vi "Verify Account Number.vi"(8 "error in":errorcluster, 11 "Module Data":T1={"UI Controls"={"ATM Messages"=refnum, "User Input"=refnum, "Right Buttons"=refnum, "Right Menu"=refnum, "Left Buttons"=refnum, "Left Menu"=refnum, "Card Simulator"=refnum, "Enter"=refnum}, "ATM Messages 2"={"Session terminate message"="Your session has been terminated\ndue to inactivity or menu selection.\nPlease take your card\n\nGoodbye!", "Welcome message"="Welcome to Acme bank.\nPlease insert your card\nand enter your account\nnumber in the User Input.\n\nPress Enter (E) when done.", "Deposit Message"="Please enter amount to deposit and press\nEnter (E) when done.", "Deposit Complete Message"="$ (Amount) Deposited", "Withdrawal Message"="Please enter amount to withdraw and press\nEnter (E) when done.", "Withdrawal Complete Message"="$ (Amount) Withdrawn", "Balance Inquiry Message"="Your Balance Is:\n$ (Balance amount from file)", "Account verification failed message"="Account information incorrect\nPlease Re-Enter Account Number.\nPress Enter (E) when done.", "Withdrawal failed message"="Insufficient funds in account\nplease check your balance\nand try again", "Card Inserted"="Card Inserted", "Main Menu message"="Welcome to Acme bank.\nFirst name, last Name (from file)\n\nplease select transaction\nby using the buttons."}, "User Input"="", "ATM Messages"="", "Acc. file path"=path "", "Accounts Data"=[], "User Input Data"={"Account No"="", "Amount"="", "Activity"=enum."Fast Cash $50"}, "Message"=""}) -> (0 "error out":errorcluster, 1 "Accounts all data":string[][](array[string]), 2 "Index account no.":i32, 3 "Is account?":bool, 4 "Balances Column":string[](array[string]))   [LabVIEW 2016]
doc: "Verify if user account exist and index account number."
uses:
  Controls/UI Controls.ctl
  Controls/ATM Messages.ctl
  Controls/Module Data.ctl
  Controls/User Input Data.ctl
  Controls/Transaction Status.ctl
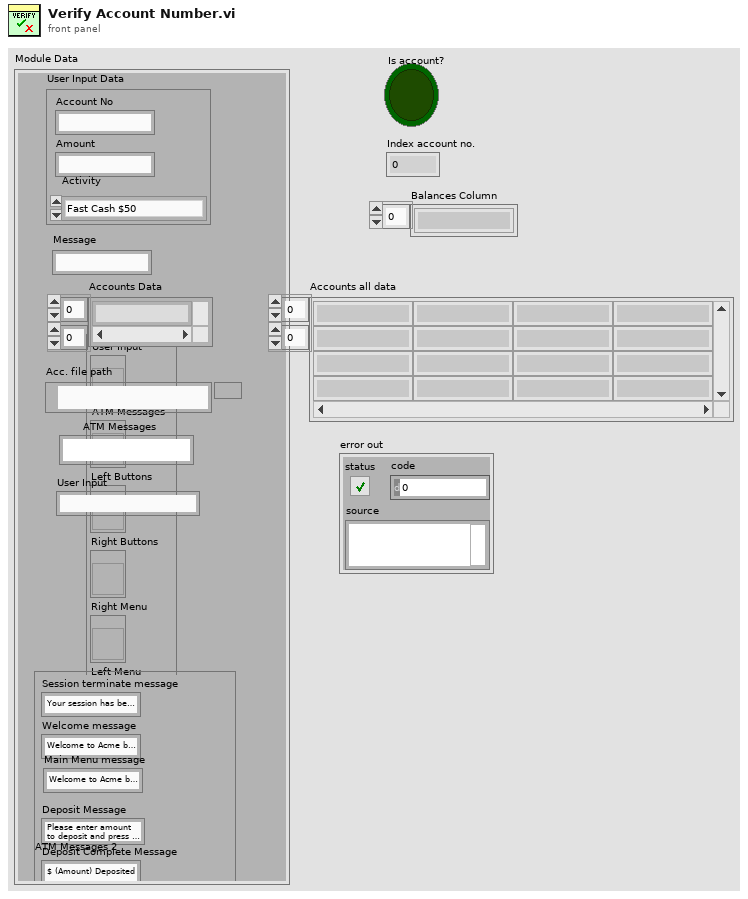
[diagram p1: front panel]
types:
  T1 = typedef "Module Data.ctl" = cluster{"UI Controls":T2, "ATM Messages 2":T3, "User Input":string, "ATM Messages":string, "Acc. file path":path, "Accounts Data":string[][], "User Input Data":T4, "Message":string}
  T2 = typedef "UI Controls.ctl" = cluster{"ATM Messages":refnum<vi>, "User Input":refnum<vi>, "Right Buttons":refnum<vi>, "Right Menu":refnum<vi>, "Left Buttons":refnum<vi>, "Left Menu":refnum<vi>, "Card Simulator":refnum<vi>, "Enter":refnum<vi>}
  T3 = typedef "ATM Messages.ctl" = cluster{"Session terminate message":string, "Welcome message":string, "Deposit Message":string, "Deposit Complete Message":string, "Withdrawal Message":string, "Withdrawal Complete Message":string, "Balance Inquiry Message":string, "Account verification failed message":string, "Withdrawal failed message":string, "Card Inserted":string, "Main Menu message":string}
  T4 = typedef "User Input Data.ctl" = cluster{"Account No":string, "Amount":string, "Activity":T5}
  T5 = typedef "Transaction Status.ctl" = enum16{"Fast Cash $50", "Withdrawal?", "Deposit?", "Account Number?"}
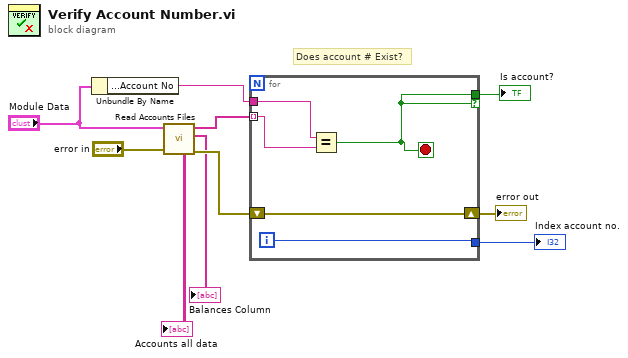
[diagram p0: block diagram]
diagram:
  # "Does account # Exist?"
  n1 = Unbundle By Name("Module Data") -> ("User Input Data.Account No"=w7:string)
  n2 = call "Read Accounts Files.vi"("error in (no error)"="error in", "Module Data"="Module Data") -> ("error out"=w4:errorcluster, "all rows"=→"Accounts all data":string[][], "Balances Column"=→"Balances Column":string[], "Acc Numbers Column"=w5:string[])  [unwired: 6 in]
  n3 = for {
    tunnel: w5 -> [w15] mode=indexing
    tunnel: [w14] -> w10 if=w14
    tunnel: w7 -> [w13]
    shift-right: [w12] -> w8
    shift-left: w4 -> [w12]
    tunnel: [w11] -> w3
    i -> [w11]
    stop <- w14 stop-if-true
    n4 = Equal?(x=w13, y=w15) -> (x = y?=w14:bool)
  }
  "Is account?" <- w10
  "error out" <- w8
  "Index account no." <- w3
